vi "RT_Comm_Manager_Enque.vi"(8 "Error In":errorcluster, 9 "Data":variant, 10 "Next State":T1, 11 "Queue In":refnum<queue>) -> (0 "Error Out":errorcluster, 3 "Queue Out":refnum<queue>)   [LabVIEW 2018]
uses:
  RT_Comm_Manager_Message.ctl
  RT_Comm_Manager_States.ctl
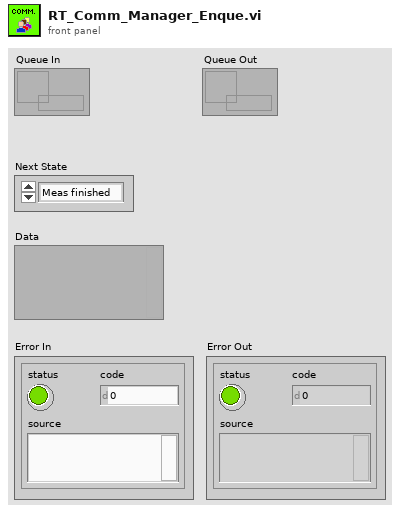
[diagram p1: front panel]
types:
  T1 = typedef "RT_Comm_Manager_States.ctl" = enum16{"Meas finished", "New connection", "Exit"}
  T2 = typedef "RT_Comm_Manager_Message.ctl" = cluster{"RT Comm Manager States":T1, "Data":variant}
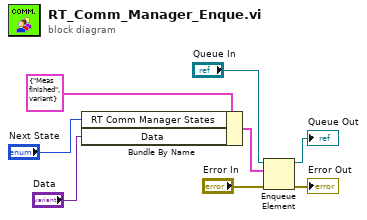
[diagram p0: block diagram]
diagram:
  n1 = Bundle By Name(cluster=T2 {"RT Comm Manager States"=enum."Meas finished", "Data"=variant} ("Connection"), "RT Comm Manager States"="Next State", "Data"="Data") -> (w3:T2)
  n2 = Enqueue Element(queue="Queue In", element=w3, error in (no error)="Error In") -> (queue out=→"Queue Out":refnum<queue>, error out=→"Error Out":errorcluster)  [unwired: 1 in, 1 out]
